vi "Remove Instrument Specifications Zeroes.vi"(8 "error in (no error)":errorcluster, 11 "INSTRUMENT CONFIGURATIONS in":T1) -> (0 "error out":errorcluster, 3 "INSTRUMENT CONFIGURATIONS out":T1)   [LabVIEW 2026, in "Settings.lvlib"]
uses:
  Settings/Settings.lvlib
  Acquisition/Instrument Specifications Configuration.ctl
  Acquisition/Instrument Specifications Cluster Configuration.ctl
  controls/UI/Measurement Role.ctl
  Acquisition/Acquisition.lvlib
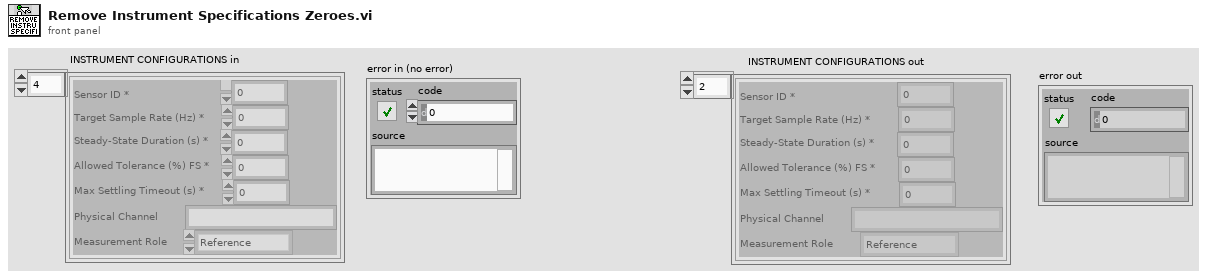
[diagram p1: front panel]
types:
  T1 = typedef "Acquisition.lvlib/Instrument Specifications Configuration.ctl" = T2[]
  T2 = typedef "Acquisition.lvlib/Instrument Specifications Cluster Configuration.ctl" = cluster{"Sensor ID *":i32, "Target Sample Rate (Hz) *":dbl, "Steady-State Duration (s) *":i32, "Allowed Tolerance (%) FS *":dbl, "Max Settling Timeout (s) *":i32, "Physical Channel":string, "Measurement Role":T3}
  T3 = typedef "Settings.lvlib/Measurement Role.ctl" = enum16{"Reference", "UUT"}
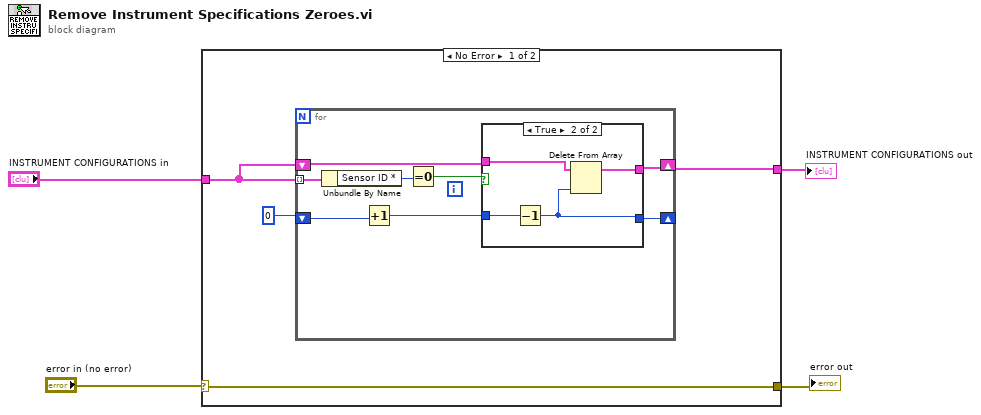
[diagram p0: block diagram]
diagram:
  n1 = case shown="No Error" "error in (no error)" {
    selector: "error in (no error)" -> [w6 w24]
    tunnel: "INSTRUMENT CONFIGURATIONS in" -> [w8 w23]
    tunnel: [w7 w23] -> w1
    tunnel: [w6 w24] -> w3
    frame No Error {
      n2 = for {
        tunnel: w8 -> [w16] mode=indexing
        shift-right: [w12] -> w7
        shift-left: w8 -> [w13]
        shift-right: [w11] -> _
        shift-left: 0 -> [w10]
        n3 = Unbundle By Name(w16) -> ("Sensor ID *"=w15:i32)
        n4 = Increment(x=w10) -> (x+1=w9:i32)
        n5 = Equal To 0?(x=w15) -> (x = 0?=w14:bool)
        n6 = case shown="True" w14 {
          tunnel: w13 -> [w18 w22]
          tunnel: [w18 w21] -> w12
          tunnel: [w17 w19] -> w11
          tunnel: w9 -> [w17 w20]
          frame False {
          }
          frame True {
            n7 = Decrement(x=w20) -> (x-1=w19:i32)
            n8 = Delete From Array(array=w22, index=w19) -> (array with subset deleted=w21:T1)  [unwired: 1 in, 1 out]
          }
        }
      }
    }
    frame Error {
    }
  }
  "error out" <- w3
  "INSTRUMENT CONFIGURATIONS out" <- w1
